vi "Command_Left_Joints.vi"(4 "Mode":enum32{"Position", "Velocity", "Effort"}(ring)=enum."Velocity", 5 "node":string, 6 "error in":errorcluster, 7 "Arm Angles (degrees)":dbl[](array[numeric])=[0.0, 0.0, 0.0, 0.0, 0.0, 0.0, 0.0]) -> (0 "error out":errorcluster, 3 "JointCommand":T1={"Mode"=enum."Position", "Arm Angles"=[-0.7853981633974483, -0.7853981633974483, 0.0, 0.7853981633974483, 0.0, 1.5707963267948966, 0.0], "Angle Names"=["left_s0", "left_s1", "left_e0", "left_e1", "left_w0", "left_w1", "left_w2"]})   [LabVIEW 2013]
uses:
  ROS/RosMessages/Clusters/JointCommand.ctl
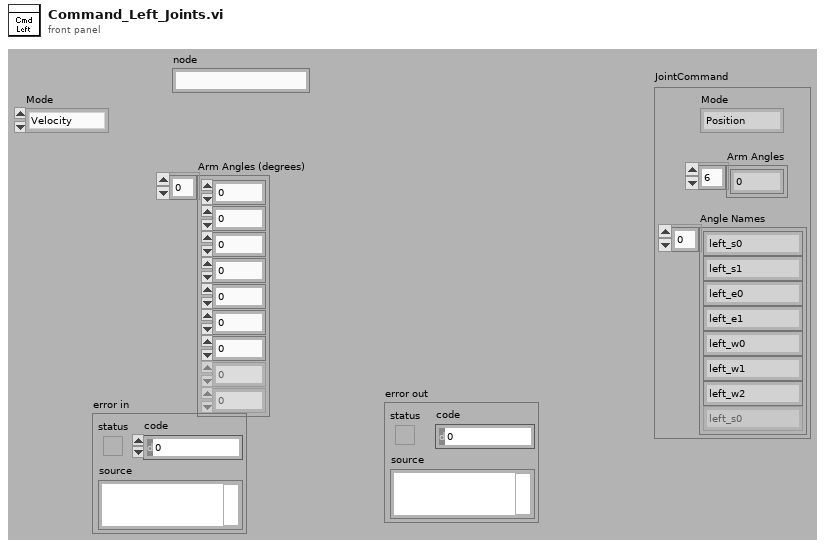
[diagram p1: front panel]
types:
  T1 = typedef "JointCommand.ctl" = cluster{"Mode":enum32{"", "Position", "Velocity", "Effort"}, "Arm Angles":dbl[], "Angle Names":string[]}
  T2 = enum16{"big-endian, network order", "native, host order", "little-endian"}
  T3 = typedef "_ROSControl.ctl" = cluster{"topic port":u16, "Node":string, "topic":string, "type":string, "node port":u32, "error ":errorcluster, "Direction":T4, "APIs":string[]}
  T4 = typedef "_ROSDirection.ctl" = enum16{"Node", "Publisher", "Subscriber", "Service Client"}
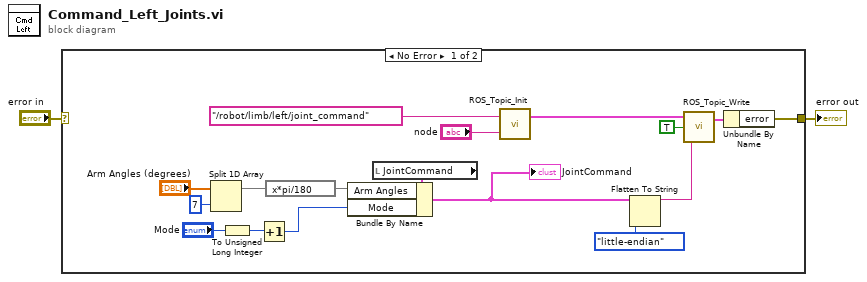
[diagram p0: block diagram]
diagram:
  n1 = case shown="No Error" "error in" {
    selector: "error in" -> [_ w20]
    tunnel: [w19 w20] -> w2
    frame No Error {
      n2 = Split 1D Array(array="Arm Angles (degrees)", index=7) -> (first subarray=w4:dbl[])  [unwired: 1 out]
      n3 = To Unsigned Long Integer(number="Mode") -> (unsigned 32bit integer=w7:u32)
      n4 = Increment(x=w7) -> (x+1=w9:u32)
      n5 = expression code="x*pi/180"(w4) -> (w8:dbl[])
      n6 = local read "JointCommand"() -> (w6:T1)
      n7 = Bundle By Name(cluster=w6, "Arm Angles"=w8, "Mode"=w9) -> (w10:T1)
      "JointCommand" <- w10
      n8 = call "ROS_Topic_Init.vi"("node"="node", "topic"="/robot/limb/left/joint_command") -> ("ROS out"=w14:T3)  [unwired: 1 in]
      n9 = Flatten To String(anything=w10, byte order (0:big-endian, network order)=T2."little-endian") -> (data string=w17:string)  [unwired: 2 in, 2 out]
      n10 = call "ROS_Topic_Write.vi"("Msg in"=w17, "Continuous?"=TRUE, "ROS in"=w14) -> ("ROS out"=w13:T3)  [unwired: 1 in]
      n11 = Unbundle By Name(w13) -> ("error"=w19:errorcluster)
    }
    frame Error {
    }
  }
  "error out" <- w2
